vi "Task 4 (copy).vi"() -> ()   [LabVIEW 2024]
panel:
  in  "T 2":dbl[](array[numeric])
  out "I":dbl[][](array[numeric])
  in  "P":dbl[][](array[numeric])
  in  "I":dbl[][](array[numeric])
  out "P-V Graph 2":cluster{"V":dbl[], "P 2":dbl[]}[](graph)
  out "I-V Graph 2":cluster{"V":dbl[], "I":dbl[]}[](graph)
  out "P":dbl[][](array[numeric])
  in  "V":dbl[](array[numeric])=[0.0, 0.1, 0.2, 0.30000000000000004, 0.4, 0.5, 0.6000000000000001, 0.7000000000000001, 0.8, 0.9, 1.0, 1.1, 1.2000000000000002, 1.3, 1.4000000000000001, 1.5, 1.6, 1.7000000000000002, 1.8, 1.9000000000000001, 2.0, 2.1, 2.2, 2.3000000000000003, 2.4000000000000004, 2.5, 2.6, 2.7, 2.8000000000000003, 2.9000000000000004, 3.0, 3.1, 3.2, 3.3000000000000003, 3.4000000000000004, 3.5, 3.6, 3.7, 3.8000000000000003, 3.9000000000000004, 4.0, 4.1000000000000005, 4.2, 4.3, 4.4, 4.5, 4.6000000000000005, 4.7, 4.800000000000001, 4.9, 5.0, 5.1000000000000005, 5.2, 5.300000000000001, 5.4, 5.5, 5.6000000000000005, 5.7, 5.800000000000001, 5.9, 6.0, 6.1000000000000005, 6.2, 6.300000000000001, 6.4, 6.5, 6.6000000000000005, 6.7, 6.800000000000001, 6.9, 7.0, 7.1000000000000005, 7.2, 7.300000000000001, 7.4, 7.5, 7.6000000000000005, 7.7, 7.800000000000001, 7.9, 8.0, 8.1, 8.200000000000001, 8.3, 8.4, 8.5, 8.6, 8.700000000000001, 8.8, 8.9, 9.0, 9.1, 9.200000000000001, 9.3, 9.4, 9.5, 9.600000000000001, 9.700000000000001, 9.8, 9.9, 10.0, 10.100000000000001, 10.200000000000001, 10.3, 10.4, 10.5, 10.600000000000001, 10.700000000000001, 10.8, 10.9, 11.0, 11.100000000000001, 11.200000000000001, 11.3, 11.4, 11.5, 11.600000000000001, 11.700000000000001, 11.8, 11.9, 12.0, 12.100000000000001, 12.200000000000001, 12.3, 12.4, 12.5, 12.600000000000001, 12.700000000000001, 12.8, 12.9, 13.0, 13.100000000000001, 13.200000000000001, 13.3, 13.4, 13.5, 13.600000000000001, 13.700000000000001, 13.8, 13.9, 14.0, 14.100000000000001, 14.200000000000001, 14.3, 14.4, 14.5, 14.600000000000001, 14.700000000000001, 14.8, 14.9, 15.0, 15.100000000000001, 15.200000000000001, 15.3, 15.4, 15.5, 15.600000000000001, 15.700000000000001, 15.8, 15.9, 16.0, 16.1, 16.2, 16.3, 16.400000000000002, 16.5, 16.6, 16.7, 16.8, 16.900000000000002, 17.0, 17.1, 17.2, 17.3, 17.400000000000002, 17.5, 17.6, 17.7, 17.8, 17.900000000000002, 18.0, 18.1, 18.2, 18.3, 18.400000000000002, 18.5, 18.6, 18.7, 18.8, 18.900000000000002, 19.0, 19.1, 19.200000000000003, 19.3, 19.400000000000002, 19.5, 19.6, 19.700000000000003, 19.8, 19.900000000000002, 20.0, 20.1, 20.200000000000003, 20.3, 20.400000000000002, 20.5, 20.6, 20.700000000000003, 20.8, 20.900000000000002, 21.0, 21.1, 21.200000000000003, 21.3, 21.400000000000002, 21.5, 21.6, 21.700000000000003, 21.8, 21.900000000000002, 22.0, 22.1, 22.200000000000003, 22.3, 22.400000000000002, 22.5, 22.6, 22.700000000000003, 22.8, 22.900000000000002, 23.0, 23.1, 23.200000000000003, 23.3, 23.400000000000002, 23.5, 23.6, 23.700000000000003, 23.8, 23.900000000000002, 24.0, 24.1, 24.200000000000003, 24.3, 24.400000000000002, 24.5, 24.6, 24.700000000000003, 24.8, 24.900000000000002, 25.0, 25.1, 25.200000000000003, 25.3, 25.400000000000002, 25.5, 25.6, 25.700000000000003, 25.8, 25.900000000000002, 26.0, 26.1, 26.200000000000003, 26.3, 26.400000000000002, 26.5, 26.6, 26.700000000000003, 26.8, 26.900000000000002, 27.0, 27.1, 27.200000000000003, 27.3, 27.400000000000002, 27.5, 27.6, 27.700000000000003, 27.8, 27.900000000000002, 28.0, 28.1, 28.200000000000003, 28.3, 28.400000000000002, 28.5, 28.6, 28.700000000000003, 28.8, 28.900000000000002, 29.0, 29.1, 29.200000000000003, 29.3, 29.400000000000002, 29.5, 29.6, 29.700000000000003, 29.8, 29.900000000000002, 30.0, 30.1, 30.200000000000003, 30.3, 30.400000000000002, 30.5, 30.6, 30.700000000000003, 30.8, 30.900000000000002, 31.0, 31.1, 31.200000000000003, 31.3, 31.400000000000002, 31.5, 31.6, 31.700000000000003, 31.8, 31.900000000000002, 32.0, 32.1, 32.2, 32.300000000000004, 32.4, 32.5, 32.6, 32.7, 32.800000000000004, 32.9, 33.0, 33.1, 33.2, 33.300000000000004, 33.4, 33.5, 33.6, 33.7, 33.800000000000004, 33.9, 34.0, 34.1, 34.2, 34.300000000000004, 34.4, 34.5, 34.6, 34.7, 34.800000000000004, 34.9, 35.0]
  in  "I_sc":dbl=8.21
  in  "G":dbl=300.0
  out "I_ph":dbl=8.2164
  in  "V_OC":dbl=32.9
  in  "N_s":dbl=54.0
  out "I_rs":dbl=1.1173361152641028e-07
  out "I_0":dbl=1.419760449337818e-07
  in  "R_s":dbl=0.221
  in  "R_sh":dbl=415.405
  out "I_sh":dbl=0.08069123942501331
  # "| Changed to control for plotting \n |\nV"
  # "Variable list"
  # "| Changed to control for plotting \n |\n |\n |\nV"
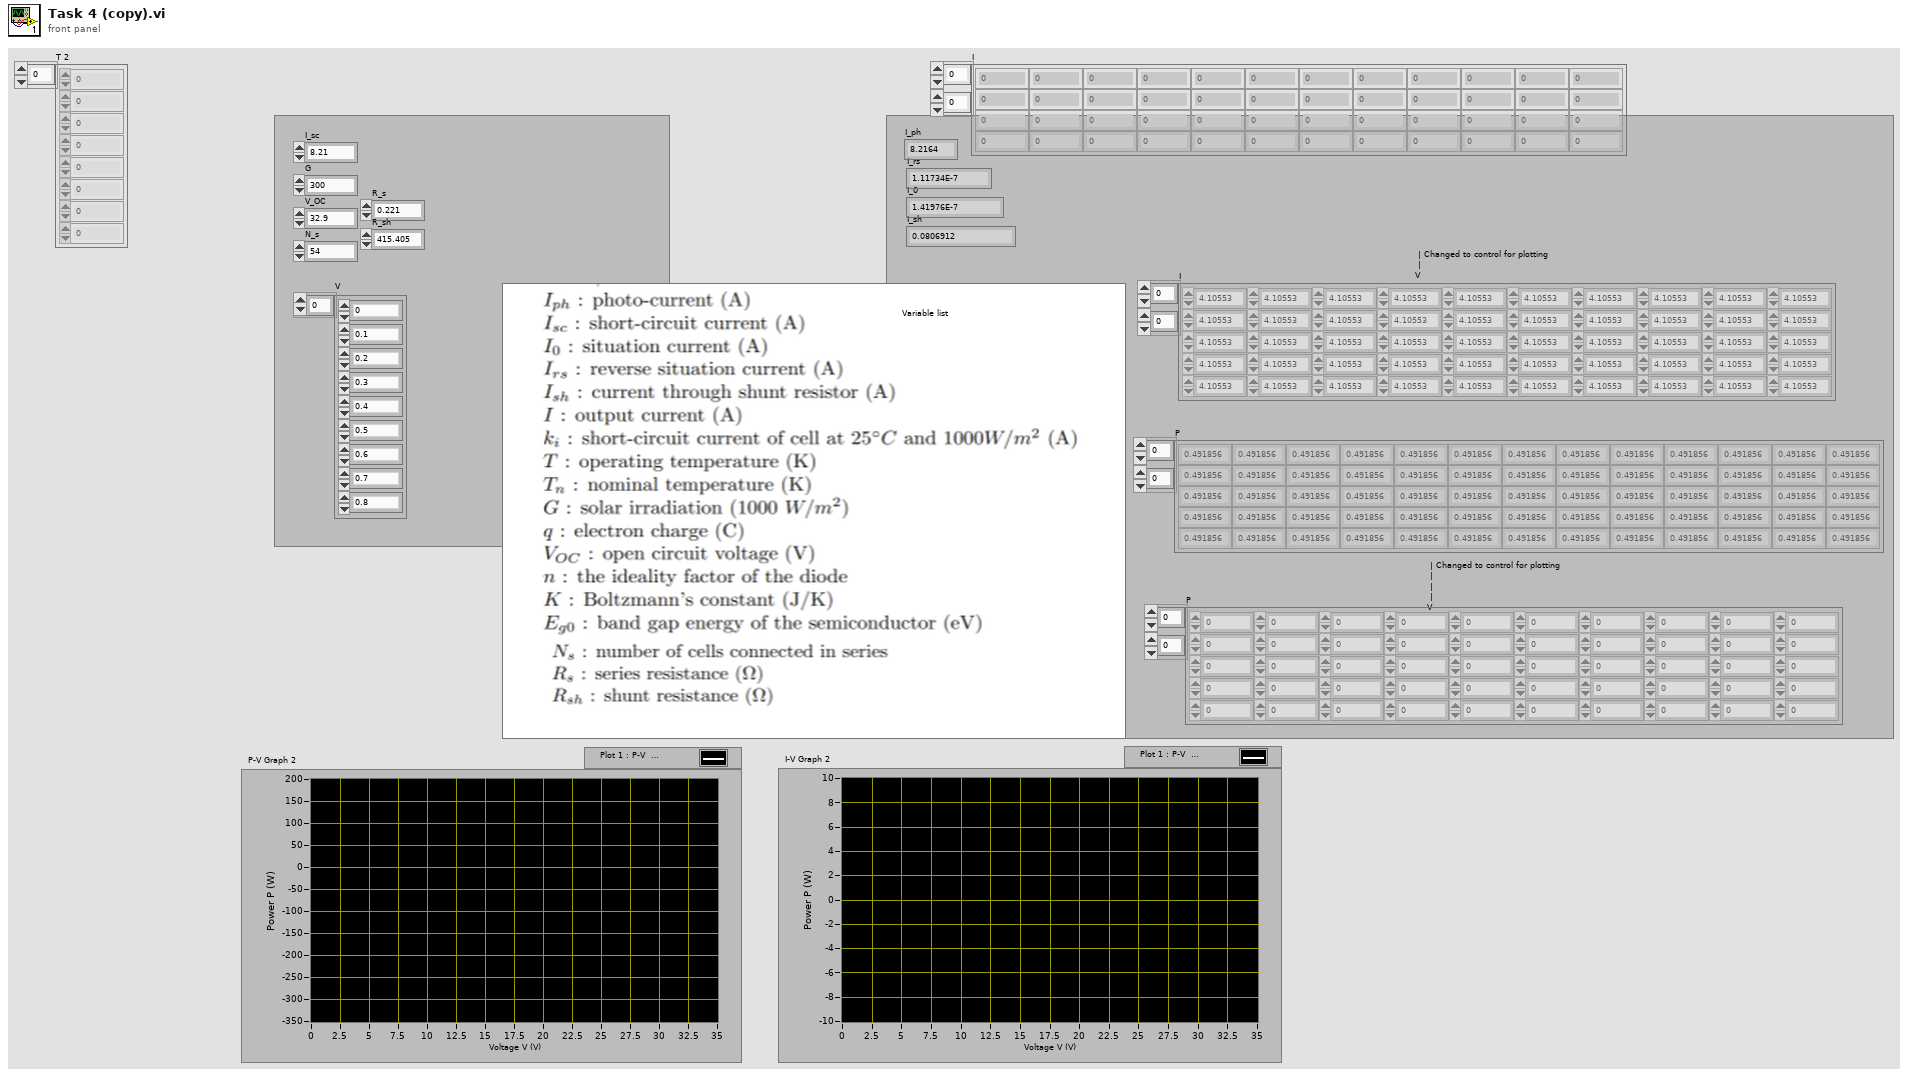
[diagram p1: front panel]
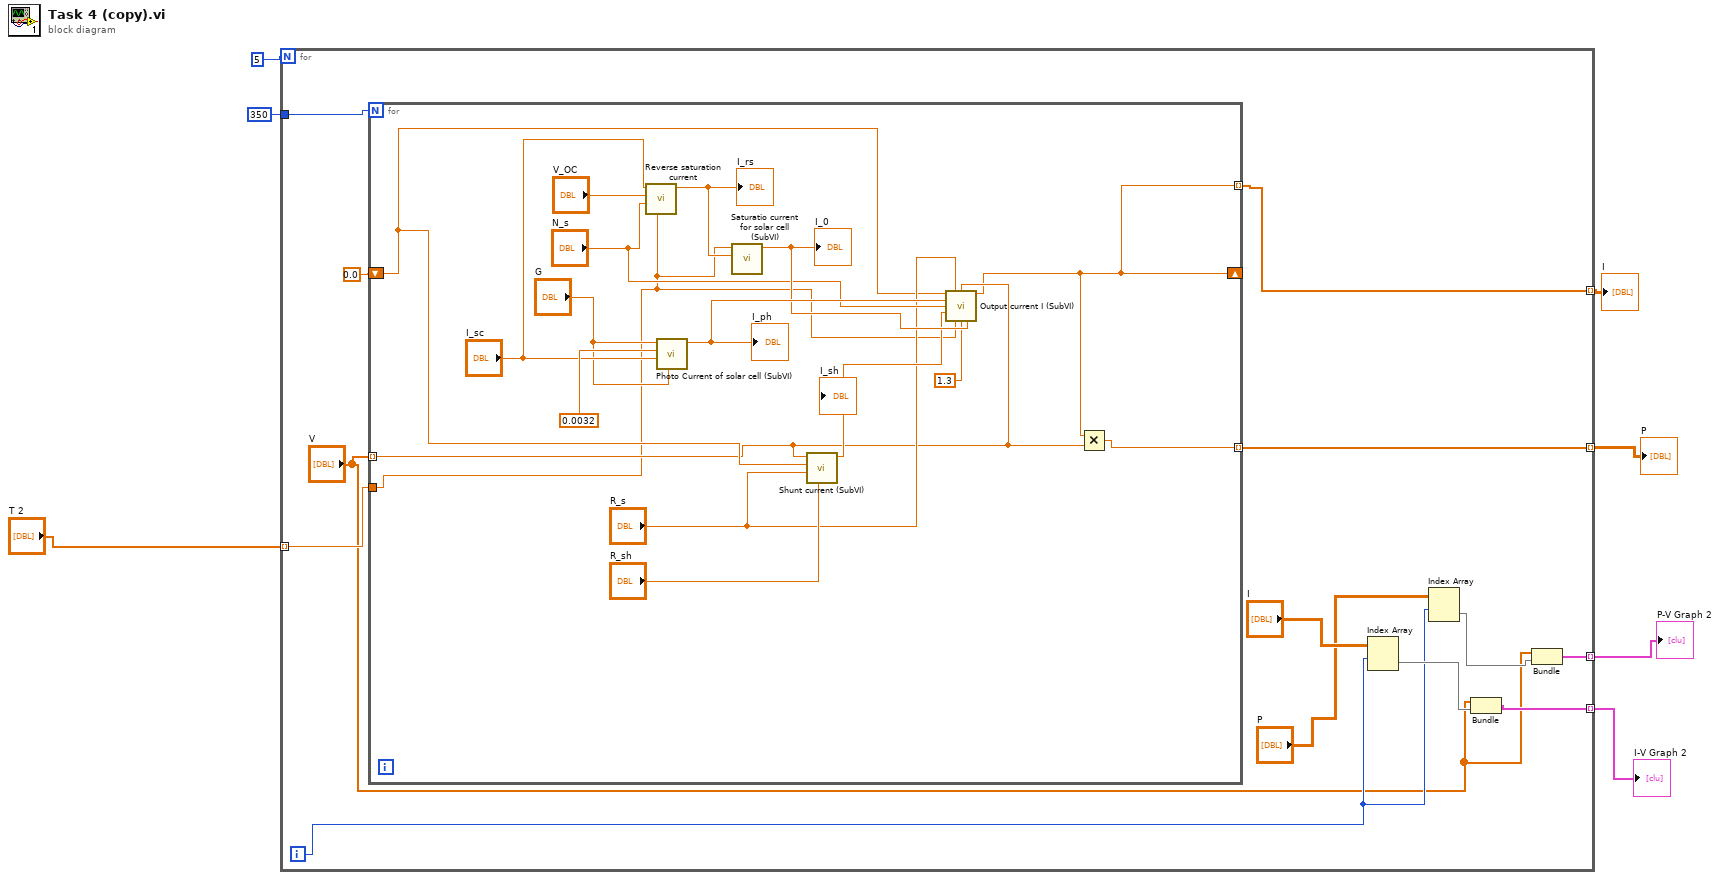
[diagram p0: block diagram]
diagram:
  n1 = for {
    N: 5 -> [_]
    tunnel: 350 -> [w19]
    tunnel: [w18] -> w2 mode=indexing
    tunnel: "T 2" -> [w17] mode=indexing
    tunnel: [w15] -> w5 mode=indexing
    tunnel: [w11] -> w4 mode=indexing
    tunnel: [w9] -> w3 mode=indexing
    i -> [w14]
    n2 = for {
      N: w19 -> [_]
      shift-right: [w23] -> _
      shift-left: 0.0 ("I") -> [w26]
      tunnel: [w23] -> w18 mode=indexing
      tunnel: "V" -> [w24] mode=indexing
      tunnel: w17 -> [w21]
      tunnel: [w25] -> w9 mode=indexing
      n3 = call "Reverse saturation current.vi"("T"=w21, "N_s"="N_s", "V_OC"="V_OC", "I_sc"="I_sc") -> ("I_rs"=w35:dbl)  [unwired: 7 in]
      "I_rs" <- w35
      n4 = call "Photo Current of solar cell (SubVI).vi"("G"="G", "I_sc"="I_sc", "k_i"=0.0032, "T"="G") -> ("I_ph"=w32:dbl)  [unwired: 7 in]
      "I_ph" <- w32
      n5 = call "Saturatio current for solar cell (SubVI).vi"("I_rs"=w35, "T"=w21) -> ("I_0"=w31:dbl)  [unwired: 9 in]
      "I_0" <- w31
      n6 = call "Shunt current (SubVI).vi"("R_sh"="R_sh", "R_s"="R_s", "I"=w26, "V"=w24) -> ("I_sh"=w30:dbl)  [unwired: 7 in]
      "I_sh" <- w30
      n7 = call "Output current I (SubVI).vi"("I_1"=w26, "R_s"="R_s", "V"=w24, "I_ph"=w32, "N_s"="N_s", "I_sh"=w30, "T"=w21, "n"=1.3, "I_0"=w31) -> ("I"=w23:dbl)  [unwired: 6 in]
      n8 = Multiply(x=w23, y=w24) -> (x*y=w25:dbl)
    }
    n9 = Index Array(array="I", index (row)=w14) -> (element=w16:dbl[])  [unwired: 1 in]
    n10 = Index Array(array="P", index (row)=w14) -> (element=w13:dbl[])  [unwired: 1 in]
    n11 = Bundle("V"="V", "I"=w16) -> (w15:cluster{"V":dbl[], "I":dbl[]})  [unwired: 1 in]
    n12 = Bundle("V"="V", "P"=w13) -> (w11:cluster{"V":dbl[], "P ":dbl[]})  [unwired: 1 in]
  }
  "I-V Graph 2" <- w5
  "P-V Graph 2" <- w4
  "P" <- w3
  "I" <- w2
